vi "DCVM Configure Range and Terminal Settings.vi"(0 "DAQmx Task In":refnum<k21>, 5 "Range and Terminal Settings":T1={"Global Settings"={"Min Range(V)"=0.0, "Max Range(V)"=0.0, "Terminal Configuration"=10083}, "Specific Channel Settings"=[]} {"Specific Channel Settings"."Terminal Configuration" items=["RSE"=10083, "NRSE"=10078, "Differential"=10106, "Pseudodifferential"=12529]; "Global Settings"."Terminal Configuration" items=["RSE"=10083, "NRSE"=10078, "Differential"=10106, "Pseudodifferential"=12529]; "Global Settings"."Max Range(V)" format="%#.2p"; "Global Settings"."Min Range(V)" format="%#.2p"}, 11 "error in (no error)":errorcluster) -> (4 "DAQmx Task Out":refnum<k21>, 15 "error out":errorcluster)   [LabVIEW 2021, in "DAQ_DC-RMS Voltage Measurement.lvlib"]
doc: "<B>Configure Range and Terminal Settings </B>\n<B>Global Settings </B>configures the range and terminal settings for all analog input voltage channels except the channels specified in the specific channel settings\n\n<B>Specific Channel Settings</B> the range and terminal settings for the physical analog input voltage channels. If the channels are specified in the list, the global settings will be applied."
uses:
  DAQ_DC-RMS Voltage Measurement.lvlib
  Typedefs/Range and Terminal Settings.ctl
  Typedefs/Specific Channel Settings.ctl
  <resource>/objmgr/daqmx.rc
panel:
  # "Min. Range(V)"
  # "Max. Range(V)"
  # "Terminal Configuration"
  # "Physical Channel Name"
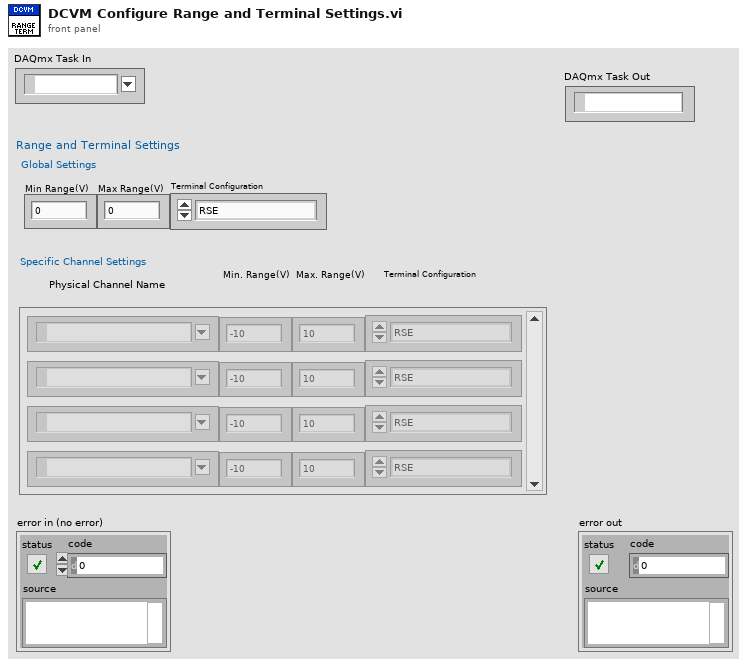
[diagram p1: front panel]
types:
  T1 = typedef "DAQ_DC-RMS Voltage Measurement.lvlib/Range and Terminal Settings.ctl" = cluster{"Global Settings":cluster{"Min Range(V)":dbl, "Max Range(V)":dbl, "Terminal Configuration":i32}, "Specific Channel Settings":T2[]}
  T2 = typedef "DAQ_DC-RMS Voltage Measurement.lvlib/Specific Channel Settings.ctl" = cluster{"Active Channels":tag, "Min Range":dbl, "Max Range":dbl, "Terminal Configuration":i32}
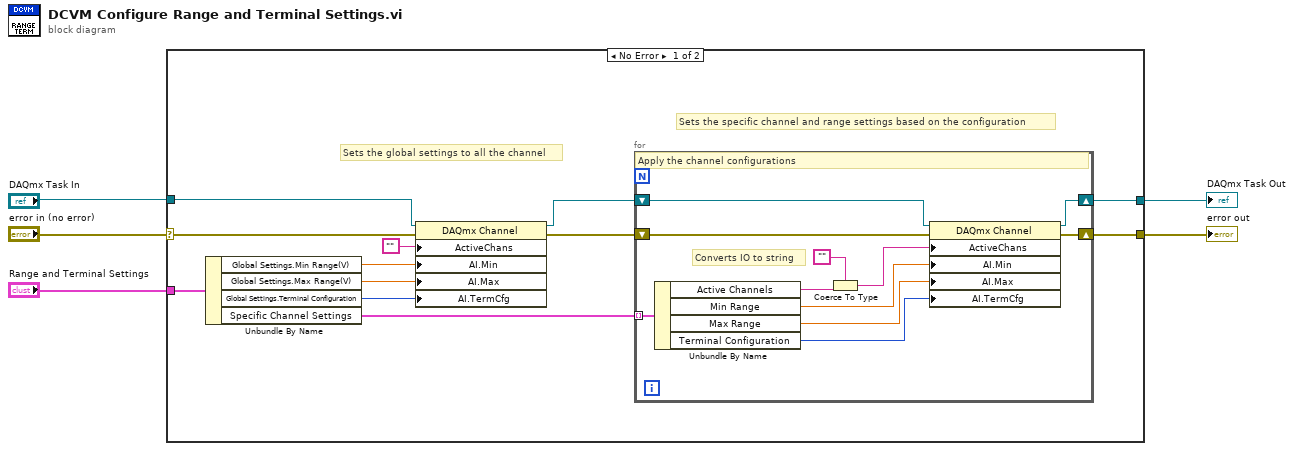
[diagram p0: block diagram]
diagram:
  n1 = case shown="No Error" "error in (no error)" {
    selector: "error in (no error)" -> [w10 w30]
    tunnel: "DAQmx Task In" -> [w12 w29]
    tunnel: "Range and Terminal Settings" -> [w8 _]
    tunnel: [w7 w29] -> w2
    tunnel: [w6 w30] -> w1
    frame No Error {
      # "Sets the specific channel and range settings based on the configuration"
      # "Sets the global settings to all the channel"
      n2 = Unbundle By Name(w8) -> ("Global Settings.Min Range(V)"=w15:dbl, "Global Settings.Max Range(V)"=w16:dbl, "Global Settings.Terminal Configuration"=w17:i32, "Specific Channel Settings"=w9:T2[])
      n3 = property class="DAQmx Channel"(reference=w12, error in=w10, "ActiveChans"="", "AI.Min"=w15, "AI.Max"=w16, "AI.TermCfg"=w17) -> (reference out=w13:refnum<k21>, error out=w11:errorcluster)
      n4 = for {
        shift-right: [w26] -> w7
        shift-left: w13 -> [w27]
        shift-right: [w28] -> w6
        shift-left: w11 -> [w21]
        tunnel: w9 -> [w24] mode=indexing
        # "Converts IO to string"
        # "Apply the channel configurations"
        n5 = Unbundle By Name(w24) -> ("Active Channels"=w19:tag, "Min Range"=w23:dbl, "Max Range"=w22:dbl, "Terminal Configuration"=w25:i32)
        n6 = Coerce To Type(0:w19, 1:"") -> (2:w18:string)
        n7 = property class="DAQmx Channel"(reference=w27, error in=w21, "ActiveChans"=w18, "AI.Min"=w23, "AI.Max"=w22, "AI.TermCfg"=w25) -> (reference out=w26:refnum<k21>, error out=w28:errorcluster)
      }
    }
    frame Error {
    }
  }
  "DAQmx Task Out" <- w2
  "error out" <- w1
